vi "Check in.vi"(8 "error in (no error)":errorcluster, 10 "data":refnum<class "Simple Class.lvclass">, 11 "reference Class in":refnum<class "Reference Class.lvclass">) -> (0 "error out":errorcluster, 3 "reference Class out":refnum<class "Reference Class.lvclass">)   [LabVIEW 2023, in "Reference Class.lvclass"]
doc: "Check in the object."
uses:
  Reference Class.lvclass
  SimpleClass/Simple Class.lvclass
  Reference Class.lvclass/Reference Class.ctl
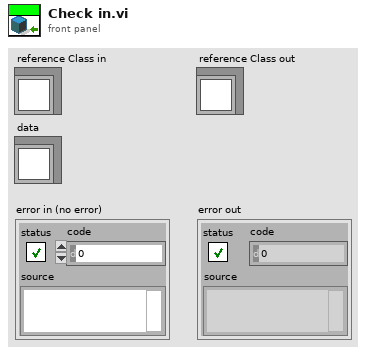
[diagram p1: front panel]
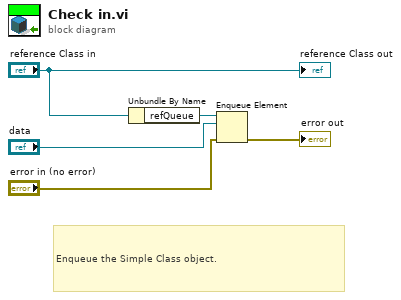
[diagram p0: block diagram]
diagram:
  # "Enqueue the Simple Class object."
  n1 = Unbundle By Name("reference Class in") -> ("refQueue"=w4:refnum<queue>)
  n2 = Enqueue Element(queue=w4, element="data", error in (no error)="error in (no error)") -> (error out=→"error out":errorcluster)  [unwired: 1 in, 2 out]
  "reference Class out" <- "reference Class in"
